vi "lib Put in Quotes.vi"(4 "String":string) -> (1 "Quoted String":string)   [LabVIEW 2021]
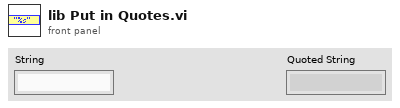
[diagram p1: front panel]
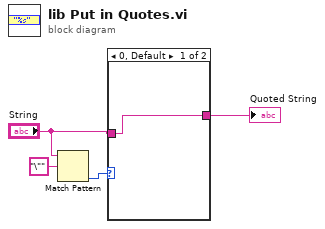
[diagram p0: block diagram]
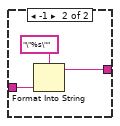
[diagram p2: hidden frame]
diagram:
  n1 = Match Pattern(string="String", regular expression="\"") -> (offset past match=w1:i32)  [unwired: 1 in, 3 out]
  n2 = case shown="0, Default" w1 {
    tunnel: [w5 w7] -> w4
    tunnel: "String" -> [w5 w6]
    frame 0, Default {
    }
    frame -1 {
      n3 = Format Into String(format string="\"%s\"", w6) -> (resulting string=w7:string)  [unwired: 2 in, 1 out]
    }
  }
  "Quoted String" <- w4
